vi "Button Do.vi"(8 "error in (no error)":errorcluster, 10 "Button Name":string, 11 "Basic Form in":refnum<class "Basic Form.lvclass">) -> (0 "error out":errorcluster, 3 "Basic Form out":refnum<class "Basic Form.lvclass">)   [LabVIEW 2020, in "Form.lvlib" / "Basic Form.lvclass"]
uses:
  Basic Form.lvclass
  Basic Form.lvclass/Basic Form.ctl
  <vilib>/Utility/miscctls.llb/LVMapReplaceAction.ctl
  Button Libraries/Button Interface Class/Button Interface.lvclass
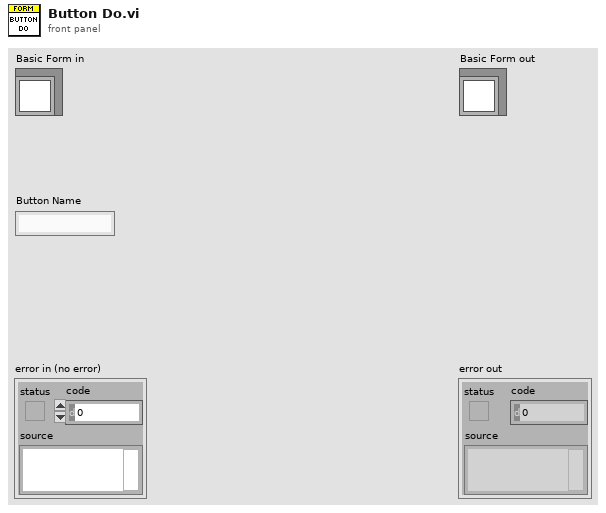
[diagram p1: front panel]
types:
  T1 = typedef "LVMapReplaceAction.ctl" = enum32{"Modify Entry only if found", "Add or Modify Entry", "Delete Entry"}
  T2 = map{string, refnum<class "Button Interface.lvclass">}
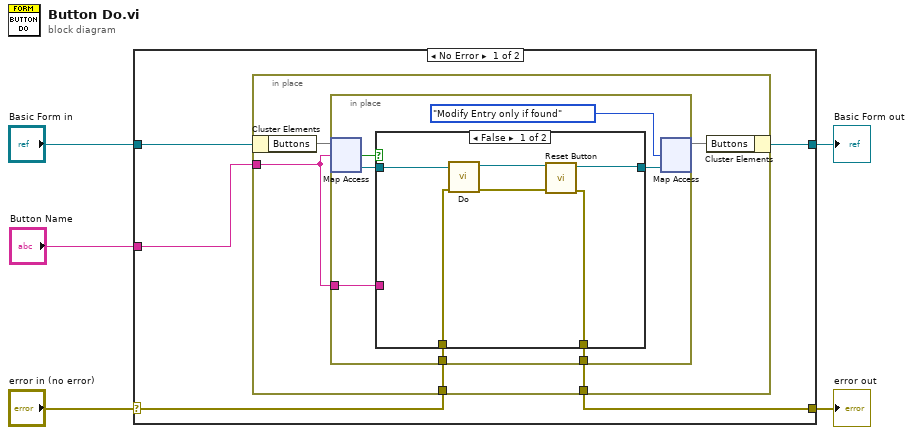
[diagram p0: block diagram]
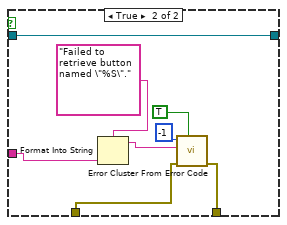
[diagram p2: hidden frame]
diagram:
  n1 = case shown="No Error" "error in (no error)" {
    selector: "error in (no error)" -> [w8 w38]
    tunnel: [w7 w38] -> w4
    tunnel: [w10 w37] -> w2
    tunnel: "Basic Form in" -> [w6 w37]
    tunnel: "Button Name" -> [w9 _]
    frame No Error {
      n2 = in-place {
        in-place-border: w9 -> [w11]
        in-place-border: w8 -> [w13]
        in-place-border: [w12] -> w7
        n3 = in-place-cluster #1(w6) -> ("Buttons"=w15:T2)
        n4 = in-place {
          in-place-border: w13 -> [w19]
          in-place-border: [w18] -> w12
          in-place-border: w11 -> [w16]
          n5 = in-place-map #2(w15, w11) -> (w21:refnum<class "Button Interface.lvclass">, w22:bool)  [unwired: 1 in]
          n6 = case shown="False" w22 {
            tunnel: w21 -> [w28 w36]
            tunnel: [w26 w36] -> w20
            tunnel: w19 -> [w24 w30]
            tunnel: [w23 w29] -> w18
            tunnel: w16 -> [_ w34]
            frame False {
              n7 = call-dynamic "Do.vi"("error in (no error)"=w24, "Button Interface in"=w28) -> ("error out"=w25:errorcluster, "Button Interface out"=w27:refnum<class "Button Interface.lvclass">)  [unwired: 8 in]
              n8 = call-dynamic "Reset Button.vi"("error in (no error)"=w25, "Button Interface in"=w27) -> ("error out"=w23:errorcluster, "Button Interface out"=w26:refnum<class "Button Interface.lvclass">)  [unwired: 8 in]
            }
            frame True {
              n9 = Format Into String(format string="Failed to retrieve button named \"%S\".", w34) -> (resulting string=w33:string)  [unwired: 2 in, 1 out]
              n10 = call <vilib>:"Error Cluster From Error Code.vi"("show call chain? (False)"=TRUE, "error in (no error)"=w30, "error message (\"\")"=w33, "error code (0)"=-1) -> ("error out"=w29:errorcluster)  [unwired: 5 in]
            }
          }
          n11 = in-place-map #2(w20, LVMapReplaceAction."Modify Entry only if found" ("action")) -> (w14:T2)  [unwired: 2 out]
        }
        n12 = in-place-cluster #1("Buttons"=w14) -> (w10:refnum<class "Basic Form.lvclass">)
      }
    }
    frame Error {
    }
  }
  "error out" <- w4
  "Basic Form out" <- w2
